vi "PhotonCamera_TakeInputSnapshot.vi"(9 "BaseNTName":string="/photonvision", 11 "CameraName":string) -> (0 "error out":errorcluster)   [LabVIEW 2019, in "PhotonVisionLib.lvlib"]
doc: "Request the camera to save a new image file from the input camera stream with overlays. Images take up space in the filesystem of the PhotonCamera. Calling it frequently will fill up disk space and eventually cause the system to stop working. Clear out images in /opt/photonvision/photonvision_config/imgSaves frequently to prevent issues.\n\nInputs:\n - cameraName -- The nickname of the camera (found in the PhotonVision UI).\n - BaseNTName - string - Base Nework Table name. (Optional. Default: /photonvision )\n\nOutputs:\n - Error Out -- Contains error information if a Network table ot other error occured."
uses:
  PhotonVisionLib.lvlib
  <vilib>/Rock Robotics/WPI/ThirdParty/JAS_Junk/TrajLib/VI/Util_GetTime_U32.vi
  <vilib>/Rock Robotics/WPI/ThirdParty/JAS_Junk/TrajLib/VI/Util_GetTime_U64.vi
  <vilib>/Rock Robotics/Network Tables/NT Read Integer.vi
  <vilib>/Rock Robotics/Network Tables/NT Write Integer.vi
  <vilib>/Rock Robotics/WPI/ThirdParty/JAS_Junk/TrajLib/Trajectory_Library.lvlib
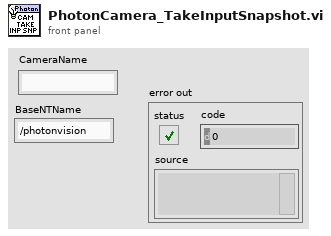
[diagram p1: front panel]
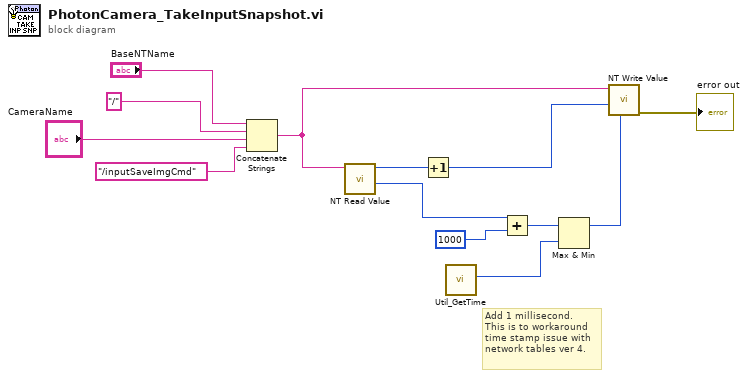
[diagram p0: block diagram]
diagram:
  # "Add 1 millisecond.\nThis is to workaround\ntime stamp issue with\nnetwork tables ver 4."
  n1 = Concatenate Strings("BaseNTName", "/", "CameraName", "/inputSaveImgCmd") -> (w10:string)
  n2 = call-poly <vilib>:"NT Read Value.vi"("name"=w10) -> ("timestamp"=w4:u64, "value"=w9:i64)  [unwired: 8 in, 1 out]
  n3 = Increment(x=w9) -> (x+1=w8:i64)
  n4 = call <vilib>:"Util_GetTime.vi"() -> ("FPGA_Time_MicroSeconds"=w5:u64)  [unwired: 9 in, 2 out]
  n5 = Add(x=w4, y=u64 1000) -> (x+y=w6:u64)
  n6 = Max & Min(x=w6, y=w5) -> (max(x,y)=w3:u64)  [unwired: 1 out]
  n7 = call-poly <vilib>:"NT Write Value.vi"("timestamp"=w3, "value"=w8, "name"=w10) -> ("error out"=→"error out":errorcluster)  [unwired: 8 in]
